vi "image_acquire_without_noise(subVI).vi"(8 "error in (no error)":errorcluster, 10 "fotogrammi mediati":i32=5, 11 "Session In":T2="cam0") -> (0 "error out":errorcluster, 3 "image out":T1(plugin-control))   [LabVIEW 2020]
doc: "Fornisce l'immagine in uscita senza rumore facendo la media di più fotogrammi selezionalibile tramite il controllo \"fotogrammi mediati\"."
uses:
  <vilib>/userdefined/High Color/IMAQdx.ctl
  <vilib>/vision/driver/NI_Vision_Acquisition_Software.lvlib
  <vilib>/vision/NI_Vision_Development_Module.lvlib
panel:
  out "input":T1(plugin-control)
  in  "stop":bool
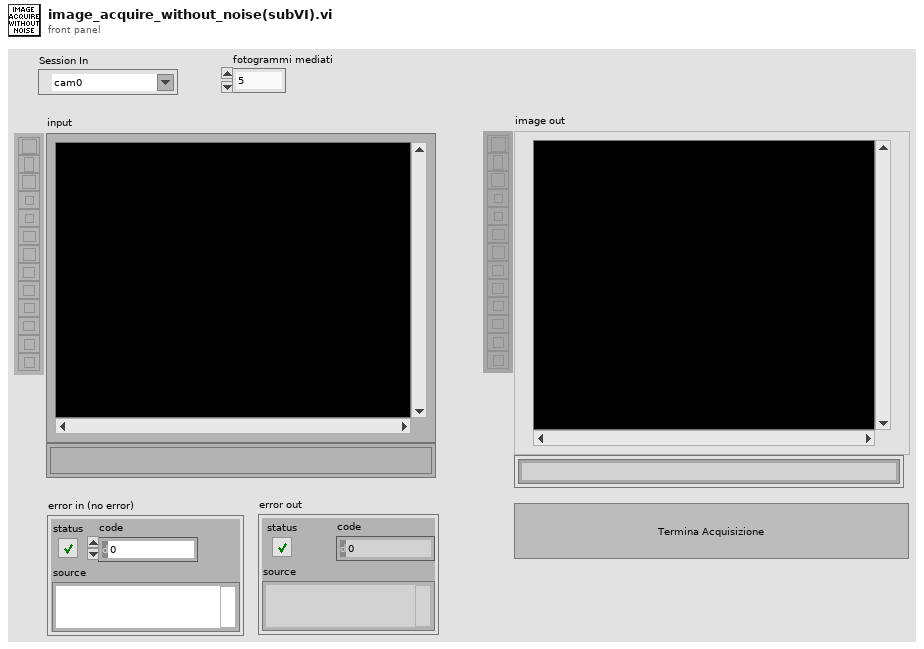
[diagram p1: front panel]
types:
  T1 = typedef "IMAQ Image.ctl" = refnum<image>
  T2 = typedef "IMAQdx.ctl" = refnum<k21>
  T3 = typedef "Image Type" = u32
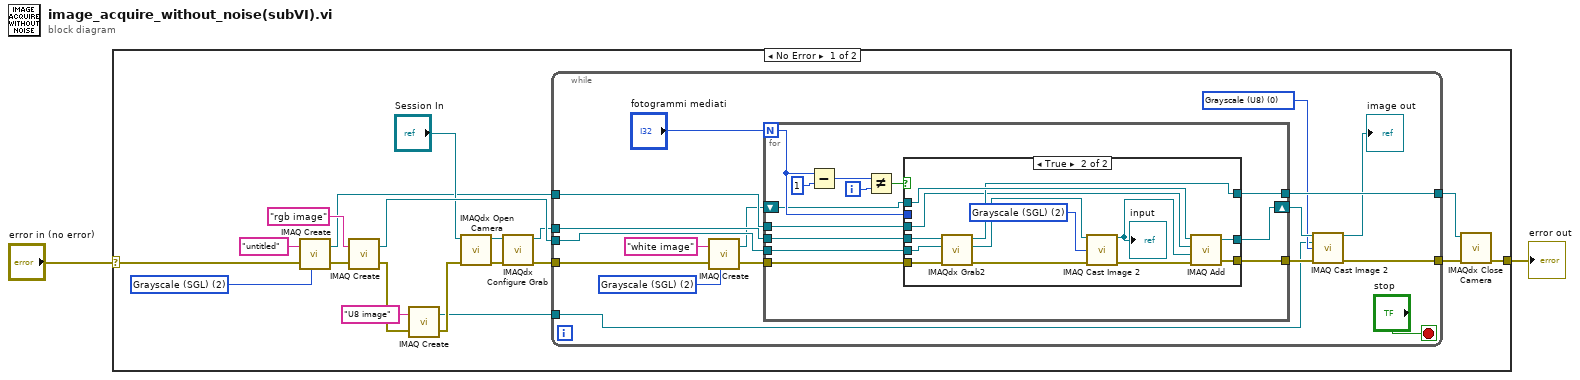
[diagram p0: block diagram]
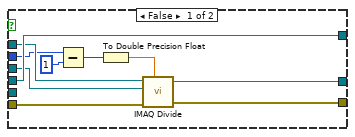
[diagram p2: hidden frame]
diagram:
  n1 = case shown="No Error" "error in (no error)" {
    selector: "error in (no error)" -> [w7 w75]
    tunnel: [w8 w75] -> w2
    frame No Error {
      w9 = T3 2 items=["Grayscale (U8)", "Grayscale (I16)", "Grayscale (SGL)", "Complex (CSG)", "RGB (U32)", "HSL (U32)", "RGB (U64)", "Grayscale (U16)"] ("Image Type")
      n2 = call "IMAQ Create"("Image Name"="untitled", "Image Type"=w9, "error in (no error)"=w7) -> ("New Image"=w12:T1, "error out"=w10:errorcluster)  [unwired: 2 in]
      n3 = call "IMAQ Create"("Image Name"="rgb image", "error in (no error)"=w10) -> ("New Image"=w18:T1, "error out"=w6:errorcluster)  [unwired: 3 in]
      n4 = call "IMAQ Create"("Image Name"="U8 image", "error in (no error)"=w6) -> ("New Image"=w3:T1, "error out"=w5:errorcluster)  [unwired: 3 in]
      n5 = call <vilib>:"IMAQdx Open Camera.vi"("error in"=w5, "Session In"="Session In") -> ("error out"=w20:errorcluster, "Session Out"=w21:T2)  [unwired: 8 in]
      n6 = call <vilib>:"IMAQdx Configure Grab.vi"("error in"=w20, "Session In"=w21) -> ("error out"=w19:errorcluster, "Session Out"=w16:T2)  [unwired: 8 in]
      n7 = while {
        tunnel: w16 -> [w37]
        tunnel: w19 -> [w30]
        tunnel: w18 -> [w38]
        tunnel: [w36] -> w15
        tunnel: [w26] -> w14
        tunnel: w12 -> [w33]
        tunnel: w3 -> [w22]
        stop <- "stop" stop-if-true
        w23 = T3 0 items=["Grayscale (U8)", "Grayscale (I16)", "Grayscale (SGL)", "Complex (CSG)", "RGB (U32)", "HSL (U32)", "RGB (U64)", "Grayscale (U16)"] ("Image Type")
        w28 = T3 2 items=["Grayscale (U8)", "Grayscale (I16)", "Grayscale (SGL)", "Complex (CSG)", "RGB (U32)", "HSL (U32)", "RGB (U64)", "Grayscale (U16)"] ("Image Type")
        n8 = call "IMAQ Create"("Image Name"="white image", "Image Type"=w28, "error in (no error)"=w30) -> ("New Image"=w32:T1, "error out"=w29:errorcluster)  [unwired: 2 in]
        n9 = for {
          N: "fotogrammi mediati" -> [w42]
          tunnel: w29 -> [w51]
          tunnel: w38 -> [w50]
          tunnel: w37 -> [w49]
          tunnel: [w48] -> w36
          tunnel: [w45] -> w27
          shift-right: [w40] -> w25
          shift-left: w32 -> [w41]
          tunnel: w33 -> [w39]
          i -> [w47]
          n10 = Subtract(x=w42, y=1) -> (x-y=w43:i32)
          n11 = Not Equal?(x=w43, y=w47) -> (x != y?=w46:bool)
          n12 = case shown="True" w46 {
            tunnel: w51 -> [w58 w72]
            tunnel: w50 -> [_ w71]
            tunnel: w49 -> [w61 w70]
            tunnel: [w61 w63] -> w48
            tunnel: [w57 w64] -> w45
            tunnel: w42 -> [w56 _]
            tunnel: w41 -> [w60 w67]
            tunnel: [w59 w66] -> w40
            tunnel: w39 -> [w52 w62]
            frame False {
              n13 = Subtract(x=w56, y=1) -> (x-y=w54:i32)
              n14 = To Double Precision Float(number=w54) -> (double precision float=w53:dbl)
              n15 = call "IMAQ Divide"("Image Src A"=w60, "Constant"=w53, "Image Dst"=w52, "error in (no error)"=w58) -> ("Image Dst Out"=w59:T1, "error out"=w57:errorcluster)  [unwired: 3 in]
            }
            frame True {
              w69 = T3 2 items=["Grayscale (U8)", "Grayscale (I16)", "Grayscale (SGL)", "Complex (CSG)", "RGB (U32)", "HSL (U32)", "RGB (U64)", "Grayscale (U16)"] ("Image Type")
              n16 = call <vilib>:"IMAQdx Grab2.vi"("error in"=w72, "Image In"=w71, "Session In"=w70) -> ("error out"=w74:errorcluster, "Image Out"=w73:T1, "Session Out"=w63:T2)  [unwired: 5 in, 1 out]
              n17 = call "IMAQ Cast Image 2"("Image Src"=w73, "Image Type"=w69, "error in (no error)"=w74) -> ("Image Dst Out"=w68:T1, "error out"=w65:errorcluster)  [unwired: 11 in]
              "input" <- w68
              n18 = call "IMAQ Add"("Image Src A"=w67, "Image Dst"=w62, "Image Src B"=w68, "error in (no error)"=w65) -> ("Image Dst Out"=w66:T1, "error out"=w64:errorcluster)  [unwired: 3 in]
            }
          }
        }
        n19 = call "IMAQ Cast Image 2"("Image Src"=w25, "Image Dst"=w22, "Image Type"=w23, "error in (no error)"=w27) -> ("Image Dst Out"=→"image out":T1, "error out"=w26:errorcluster)  [unwired: 10 in]
      }
      n20 = call <vilib>:"IMAQdx Close Camera.vi"("error in"=w14, "Session In"=w15) -> ("error out"=w8:errorcluster)  [unwired: 9 in]
    }
    frame Error {
    }
  }
  "error out" <- w2
